vi "Word_Insert_Picture.vi"(0 "Word.Document":refnum<k7>, 1 "Word.InlineShapes":refnum<k7>, 2 "alignment (default)":T1, 5 "Image file path":string, 7 "Start":i32, 9 "End":i32, 11 "error in (no error)":errorcluster, 12 "Insertion point":u16(ring)=1 items=["begining of document", "end of document", "bookmark", "Custom"], 13 "bookmark name":string) -> (8 "Start out":i32, 10 "End out":i32, 15 "error out 2":errorcluster)   [LabVIEW 2017, in "NI_ReportGenerationToolkit.lvlib"]
uses:
  <vilib>/addons/_office/NI_ReportGenerationToolkit.lvlib
  <vilib>/Utility/NIReport.llb/HTML Report Image Alignment.ctl
  <vilib>/Utility/NIReport.llb/NI_ReportGenerationCore.lvlib
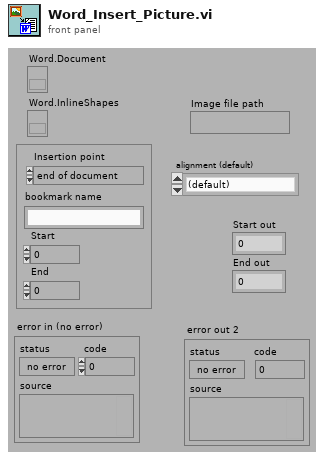
[diagram p1: front panel]
types:
  T1 = typedef "NI_ReportGenerationCore.lvlib/HTML Report Image Alignment.ctl" = enum16{"(default)", "LEFT", "RIGHT", "TOP", "TEXTTOP", "MIDDLE", "ABSMIDDLE", "BASELINE", "BOTTOM", "ABSBOTTOM"}
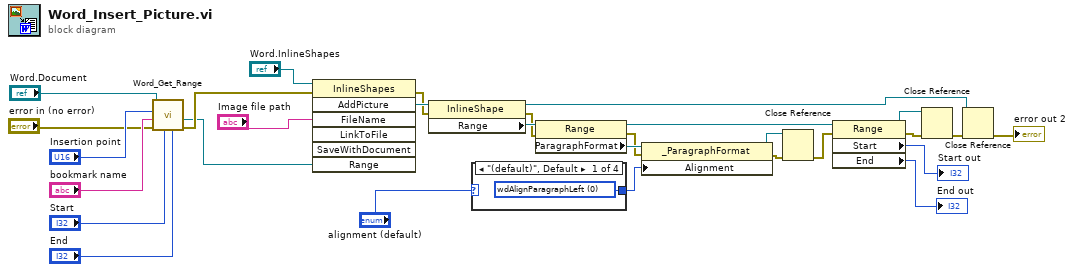
[diagram p0: block diagram]
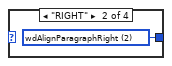
[diagram p2: hidden frame]
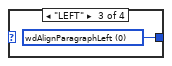
[diagram p3: hidden frame]
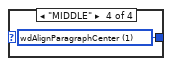
[diagram p4: hidden frame]
diagram:
  n1 = call <vilib>:"Word_Get_Range.vi"("end"="End", "start"="Start", "error in"="error in (no error)", "bookmark name"="bookmark name", "insertion point"="Insertion point", "document in"="Word.Document") -> ("error out (no error)"=w26:errorcluster, "range"=w17:refnum<k7>)  [unwired: 4 out]
  n2 = invoke class="InlineShapes" method="AddPicture"(reference="Word.InlineShapes", error in=w26, "FileName"="Image file path", "Range"=w17) -> (error out=w8:errorcluster, "AddPicture"=w20:refnum<k7>)  [unwired: 3 in, 5 out]
  n3 = property class="InlineShape"(reference=w20, error in=w8) -> (reference out=w10:refnum<k7>, error out=w9:errorcluster, "Range"=w19:refnum<k7>)
  n4 = case shown="\"(default)\", Default" "alignment (default)" {
    tunnel: [w30 w31 w32 w33] -> w5
    frame "(default)", Default {
      w30 = 0 items=["wdAlignParagraphLeft"=0, "wdAlignParagraphCenter"=1, "wdAlignParagraphRight"=2, "wdAlignParagraphJustify"=3, "wdAlignParagraphDistribute"=4, "wdAlignParagraphJustifyMed"=5, "wdAlignParagraphJustifyHi"=7, "wdAlignParagraphJustifyLow"=8] ("Alignment")
    }
    frame "RIGHT" {
      w31 = 2 items=["wdAlignParagraphLeft"=0, "wdAlignParagraphCenter"=1, "wdAlignParagraphRight"=2, "wdAlignParagraphJustify"=3, "wdAlignParagraphDistribute"=4, "wdAlignParagraphJustifyMed"=5, "wdAlignParagraphJustifyHi"=7, "wdAlignParagraphJustifyLow"=8] ("Alignment")
    }
    frame "LEFT" {
      w32 = 0 items=["wdAlignParagraphLeft"=0, "wdAlignParagraphCenter"=1, "wdAlignParagraphRight"=2, "wdAlignParagraphJustify"=3, "wdAlignParagraphDistribute"=4, "wdAlignParagraphJustifyMed"=5, "wdAlignParagraphJustifyHi"=7, "wdAlignParagraphJustifyLow"=8] ("Alignment")
    }
    frame "MIDDLE" {
      w33 = 1 items=["wdAlignParagraphLeft"=0, "wdAlignParagraphCenter"=1, "wdAlignParagraphRight"=2, "wdAlignParagraphJustify"=3, "wdAlignParagraphDistribute"=4, "wdAlignParagraphJustifyMed"=5, "wdAlignParagraphJustifyHi"=7, "wdAlignParagraphJustifyLow"=8] ("Alignment")
    }
  }
  n5 = property class="Range"(reference=w19, error in=w9) -> (reference out=w16:refnum<k7>, error out=w7:errorcluster, "ParagraphFormat"=w18:refnum<k7>)
  n6 = property class="_ParagraphFormat"(reference=w18, error in=w7, "Alignment"=w5) -> (reference out=w11:refnum<k7>, error out=w15:errorcluster)
  n7 = Close Reference(reference=w11, error in (no error)=w15) -> (error out=w13:errorcluster)
  n8 = property class="Range"(reference=w16, error in=w13) -> (reference out=w1:refnum<k7>, error out=w2:errorcluster, "Start"=→"Start out":i32, "End"=→"End out":i32)
  n9 = Close Reference(reference=w1, error in (no error)=w2) -> (error out=w14:errorcluster)
  n10 = Close Reference(reference=w10, error in (no error)=w14) -> (error out=→"error out 2":errorcluster)
